vi "Set_Home_Position.vi"(8 "Error In":errorcluster, 9 "Home Position":i64, 10 "Node":u8, 11 "Serial In":refnum<visa-resource-name>) -> (0 "Error Out":errorcluster, 3 "Serial Out":refnum<visa-resource-name>)   [LabVIEW 2019]
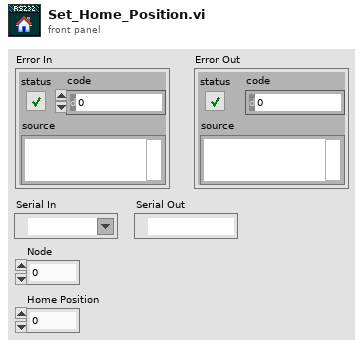
[diagram p1: front panel]
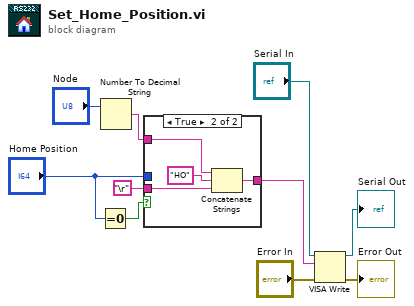
[diagram p0: block diagram]
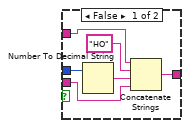
[diagram p2: hidden frame]
diagram:
  n1 = Equal To 0?(x="Home Position") -> (x = 0?=w1:bool)
  n2 = Number To Decimal String(number="Node") -> (decimal integer string=w4:string)  [unwired: 1 in]
  n3 = case shown="True" w1 {
    tunnel: "Home Position" -> [w16 _]
    tunnel: "\r" -> [w15 w17]
    tunnel: w4 -> [w14 w20]
    tunnel: [w12 w19] -> w3
    frame False {
      n4 = Number To Decimal String(number=w16) -> (decimal integer string=w13:string)  [unwired: 1 in]
      n5 = Concatenate Strings(w14, "HO" ("string"), w13, w15) -> (w12:string)
    }
    frame True {
      n6 = Concatenate Strings(w20, "HO" ("string"), w17) -> (w19:string)
    }
  }
  n7 = VISA Write(VISA resource name="Serial In", write buffer=w3, error in (no error)="Error In") -> (VISA resource name out=→"Serial Out":refnum<visa-resource-name>, error out=→"Error Out":errorcluster)  [unwired: 1 out]
